vi "Query Multi Eval Meas List Segment Bandwidth Part.vi"(0 "VISA resource name":refnum<visa-resource-name>, 1 "BWP (0)":i32, 5 "Instance (1)":T2=1, 7 "Segment (1)":i32=1, 9 "CC (1)":T1=1, 11 "error in (no error)":errorcluster) -> (4 "VISA resource name out":refnum<visa-resource-name>, 6 "Subcarrier Spacing":i32, 8 "Cyclic Prefix":i32, 10 "Number RB":i32, 14 "Start RB":i32, 15 "error out":errorcluster)   [LabVIEW 2020, in "Rohde&Schwarz CMWXP NR FR1 Measurement.lvlib"]
doc: "Queries basic properties of the <BWP> on carrier <cc> in segment <no>.\n\nAttribute:\n-\n\nRemote-control command:\nCONFigure:NRSub:MEAS<i>:LIST:SEGMent<no>[:CC<cc>]:BWPart?"
uses:
  <instrlib>/Rohde&Schwarz CMWXP NR FR1 Measurement/Rohde&Schwarz CMWXP NR FR1 Measurement.lvlib
  <instrlib>/Rohde&Schwarz CMWXP NR FR1 Measurement/Private/_Instance.ctl
  <instrlib>/Rohde&Schwarz CMWXP NR FR1 Measurement/Private/_Carrier Component.ctl
  <instrlib>/Rohde&Schwarz CMWXP NR FR1 Measurement/Private/rsidr_core.llb/rsidr_core.lvlib
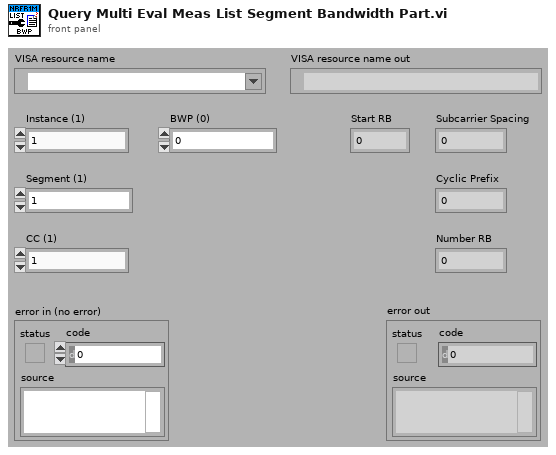
[diagram p1: front panel]
types:
  T1 = typedef "Rohde&Schwarz CMWXP NR FR1 Measurement.lvlib/_Carrier Component.ctl" = i32
  T2 = typedef "Rohde&Schwarz CMWXP NR FR1 Measurement.lvlib/_Instance.ctl" = i32
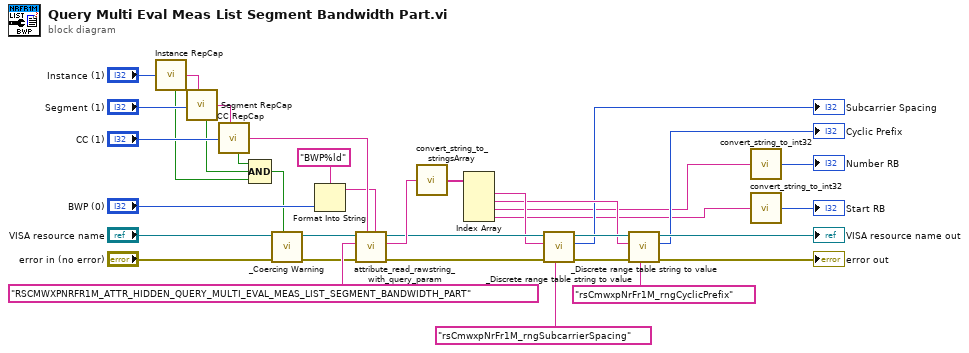
[diagram p0: block diagram]
diagram:
  n1 = call <instrlib>:"Instance RepCap.vi"("Instance In"="Instance (1)") -> ("In Range?"=w4:bool, "RepCap Identifier Out"=w33:string)  [unwired: 1 in]
  n2 = call <instrlib>:"Segment RepCap.vi"("Segment In"="Segment (1)", "RepCap String In (\"\")"=w33) -> ("In Range?"=w3:bool, "RepCap Identifier Out"=w35:string)
  n3 = call <instrlib>:"CC RepCap.vi"("CC In"="CC (1)", "RepCap String In (\"\")"=w35) -> ("In Range?"=w1:bool, "RepCap Identifier Out"=w31:string)
  n4 = Compound Arithmetic op=AND(w1, w3, w4) -> (w2:bool)
  n5 = call <instrlib>:"_Coercing Warning.vi"("In Range?"=w2, "error in (no error)"="error in (no error)", "VISA resource name"="VISA resource name") -> ("error out"=w6:errorcluster, "VISA resource name out"=w5:refnum<visa-resource-name>)  [unwired: 7 in]
  n6 = Format Into String(format string="BWP%ld", "BWP (0)") -> (resulting string=w28:string)  [unwired: 2 in, 1 out]
  n7 = call <instrlib>:"attribute_read_rawstring_with_query_param.vi"("Query Parameter (None)"=w28, "Repeated Capability"=w31, "error in"=w6, "Attribute ID"="RSCMWXPNRFR1M_ATTR_HIDDEN_QUERY_MULTI_EVAL_MEAS_LIST_SEGMENT_BANDWIDTH_PART", "VISA resource name"=w5) -> ("error out"=w24:errorcluster, "Raw String out"=w26:string, "VISA resource name out"=w23:refnum<visa-resource-name>)  [unwired: 4 in]
  n8 = call <instrlib>:"convert_string_to_stringsArray.vi"("String in"=w26) -> ("string array out"=w25:string[])  [unwired: 3 in, 1 out]
  n9 = Index Array(array=w25) -> (element #1=w20:string, element #2=w19:string, element #3=w12:string, element #4=w10:string)  [unwired: 4 in]
  n10 = call <instrlib>:"_Discrete range table string to value.vi"("Discrete Range Table Identifier"="rsCmwxpNrFr1M_rngSubcarrierSpacing", "error in (no error)"=w24, "String Value In"=w20, "VISA resource name"=w23) -> ("error out"=w22:errorcluster, "Enum Value"=→"Subcarrier Spacing":i32, "VISA resource name out"=w21:refnum<visa-resource-name>)  [unwired: 5 in]
  n11 = call <instrlib>:"_Discrete range table string to value.vi"("Discrete Range Table Identifier"="rsCmwxpNrFr1M_rngCyclicPrefix", "error in (no error)"=w22, "String Value In"=w19, "VISA resource name"=w21) -> ("error out"=→"error out":errorcluster, "Enum Value"=→"Cyclic Prefix":i32, "VISA resource name out"=→"VISA resource name out":refnum<visa-resource-name>)  [unwired: 5 in]
  n12 = call <instrlib>:"convert_string_to_int32.vi"("String in"=w12) -> ("int32 value out"=→"Number RB":i32)  [unwired: 4 in]
  n13 = call <instrlib>:"convert_string_to_int32.vi"("String in"=w10) -> ("int32 value out"=→"Start RB":i32)  [unwired: 4 in]
